vi "DHE_SetConfigFile.vi"(2 "DHE_ConfigFile":path) -> ()   [LabVIEW 2016]
uses:
  private/vis/DHE_GBLDriverVariables.vi
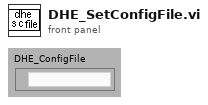
[diagram p1: front panel]
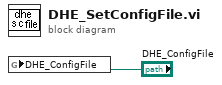
[diagram p0: block diagram]
diagram:
  n1 = global write "DHE_GBLDriverVariables.vi" "DHE_ConfigFile"("DHE_ConfigFile") -> ()
